vi "_DeleteUser.vi"(8 "error in":errorcluster, 10 "User":T1={"UserName"="", "Password"="", "Role"=enum."Admin"}, 11 "User List":T1[](array[typedef])) -> (0 "error out":errorcluster, 3 "User List":T1[](array[typedef]))   [LabVIEW 2017, in "Login-UI.lvlib"]
uses:
  Login-UI.lvlib
  User-Info.ctl
  User-Role.ctl
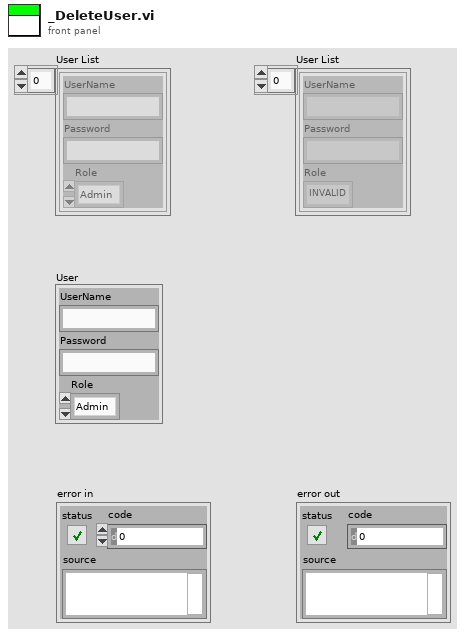
[diagram p1: front panel]
types:
  T1 = typedef "Login-UI.lvlib/User-Info.ctl" = cluster{"UserName":string, "Password":string, "Role":T2}
  T2 = typedef "Login-UI.lvlib/User-Role.ctl" = enum16{"INVALID", "Operator", "Engineer", "Admin"}
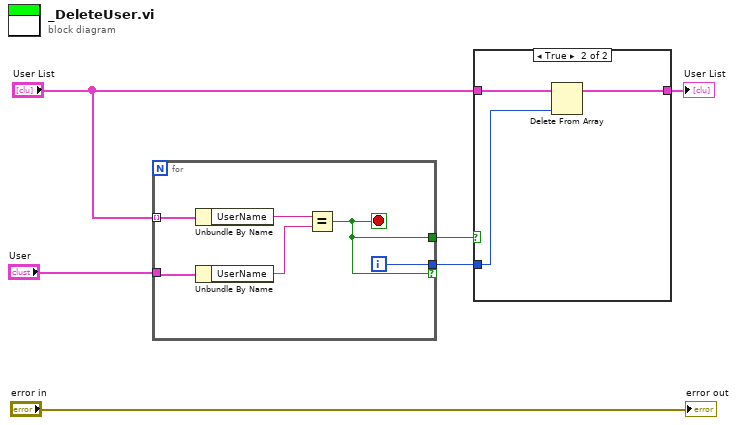
[diagram p0: block diagram]
diagram:
  n1 = for {
    tunnel: "User List" -> [w12] mode=indexing
    tunnel: "User" -> [w10]
    tunnel: [w8] -> w3 if=w7
    tunnel: [w7] -> w5
    i -> [w8]
    stop <- w7 stop-if-true
    n2 = Unbundle By Name(w12) -> ("UserName"=w11:string)
    n3 = Unbundle By Name(w10) -> ("UserName"=w9:string)
    n4 = Equal?(x=w11, y=w9) -> (x = y?=w7:bool)
  }
  n5 = case shown="True" w5 {
    tunnel: "User List" -> [w13 w16]
    tunnel: w3 -> [_ w14]
    tunnel: [w13 w15] -> w2
    frame False {
    }
    frame True {
      n6 = Delete From Array(array=w16, index=w14) -> (array with subset deleted=w15:T1[])  [unwired: 1 in, 1 out]
    }
  }
  "User List" <- w2
  "error out" <- "error in"
